vi "hwOperation_Tree.vi"   [LabVIEW 2016]
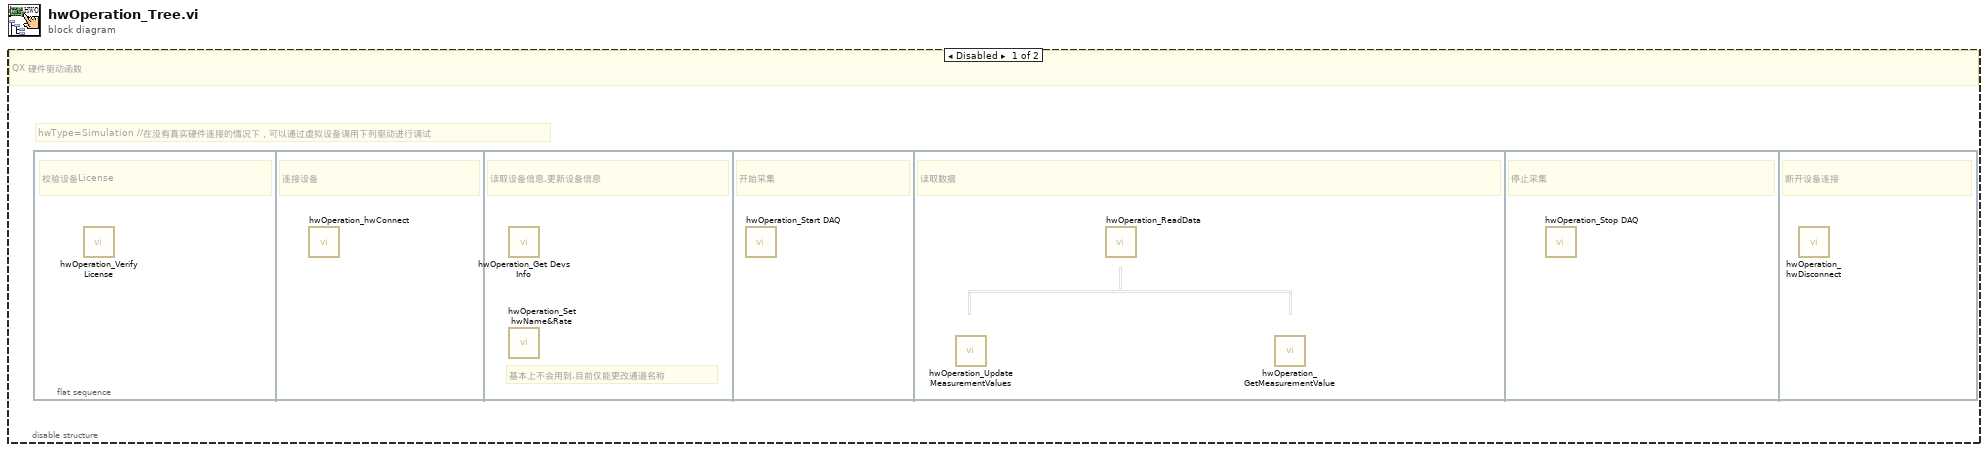
[diagram p0: block diagram]
diagram:
  n1 = disable-structure shown="Disabled" {
    frame Disabled {
      # "hwType=Simulation //在没有真实硬件连接的情况下，可以通过虚拟设备调用下列驱动进行调试"
      # "QX 硬件驱动函数"
      n2 = flat-sequence {
        frame #0 {
          # "校验设备License"
          n3 = call "hwOperation_Verify License.vi"() -> ()  [unwired: 11 in, 1 out]
        }
        frame #1 {
          # "连接设备"
          n4 = call "hwOperation_hwConnect.vi"() -> ()  [unwired: 9 in, 3 out]
        }
        frame #2 {
          # "基本上不会用到,目前仅能更改通道名称"
          # "读取设备信息,更新设备信息"
          n5 = call "hwOperation_Get Devs Info.vi"() -> ()  [unwired: 9 in, 3 out]
          n6 = call "hwOperation_Set hwName&Rate.vi"() -> ()  [unwired: 9 in, 3 out]
        }
        frame #3 {
          # "开始采集"
          n7 = call "hwOperation_Start DAQ.vi"() -> ()  [unwired: 9 in, 3 out]
        }
        frame #4 {
          # "读取数据"
          n8 = call "hwOperation_Update MeasurementValues.vi"() -> ()  [unwired: 10 in, 2 out]
          n9 = call "hwOperation_ReadData.vi"() -> ()  [unwired: 8 in, 4 out]
          n10 = call "hwOperation_GetMeasurementValue.vi"() -> ()  [unwired: 6 in, 6 out]
        }
        frame #5 {
          # "停止采集"
          n11 = call "hwOperation_Stop DAQ.vi"() -> ()  [unwired: 10 in, 2 out]
        }
        frame #6 {
          # "断开设备连接"
          n12 = call "hwOperation_hwDisconnect.vi"() -> ()  [unwired: 10 in, 2 out]
        }
      }
    }
    frame Enabled {
    }
  }
